vi "Write txt.vi"(8 "error in":errorcluster, 11 "IN String":string) -> (0 "error out":errorcluster, 3 "out":string)   [LabVIEW 2009]
uses:
  Global/Global 1.vi
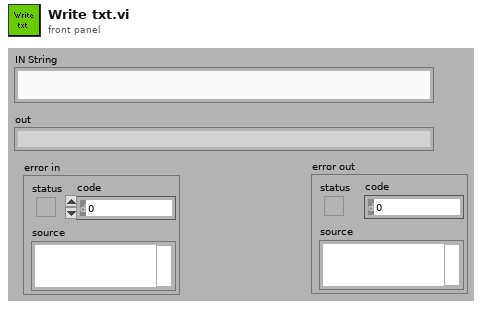
[diagram p1: front panel]
types:
  T1 = enum16{"open", "replace", "create", "open or create", "replace or create", "replace or create with confirmation"}
  T2 = cluster{"serial number":string, "Part number":string, "Revision letter ":string, "Revision counter":string, "Manufature":string, "Year Week":string}
  T3 = cluster{".128 file":path, "Appliction firmware file":path, "Data file":path, "Txt path":path, "EXCEL path":path}
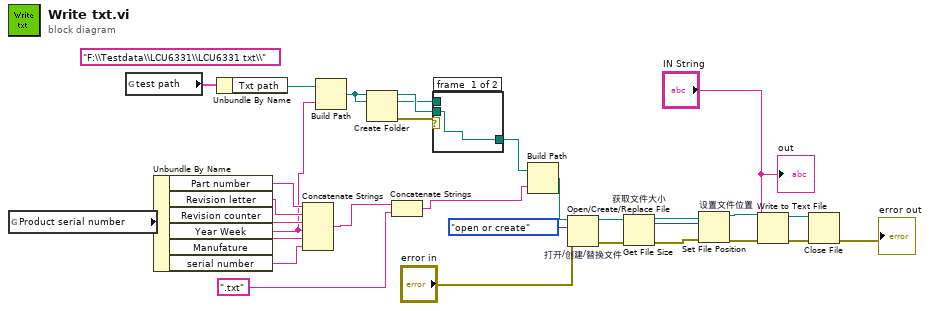
[diagram p0: block diagram]
diagram:
  (unwired) "F:\\Testdata\\LCU6331\\LCU6331 txt\\" ("string")
  n1 = global read "Global 1.vi" "Product serial number"() -> (w16:T2)
  n2 = global read "Global 1.vi" "test path"() -> (w2:T3)
  n3 = Unbundle By Name(w16) -> ("Part number"=w15:string, "Revision letter"=w14:string, "Revision counter"=w13:string, "Year Week"=w9:string, "Manufature"=w12:string, "serial number"=w11:string)
  n4 = Unbundle By Name(w2) -> ("Txt path"=w1:path)
  n5 = Concatenate Strings(w15, w14, w13, w9, w12, w11) -> (w10:string)
  n6 = Build Path(base path=w1, name or relative path=w9) -> (appended path=w6:path)
  n7 = Create Folder(path (use dialog)=w6) -> (created path=w8:path, error out=w7:errorcluster)  [unwired: 1 in, 2 out]
  n8 = Concatenate Strings(w10, ".txt") -> (w4:string)
  n9 = case shown="Error" w7 {
    tunnel: w8 -> [w31 _]
    tunnel: [w31 w32] -> w5
    tunnel: w6 -> [_ w32]
    frame #0 {
    }
    frame #1 {
    }
  }
  n10 = Build Path(base path=w5, name or relative path=w4) -> (appended path=w3:path)
  n11 = Open/Create/Replace File "打开/创建/替换文件"(file path (use dialog)=w3, error in="error in", operation (0:open)=T1."open or create" ("操作(0:open)")) -> (refnum out=w27:refnum<file>, error out=w25:errorcluster)  [unwired: 4 out]
  n12 = Get File Size "获取文件大小"(file=w27, error in=w25) -> (refnum out=w28:refnum<file>, size (in bytes)=w22:i64, 0:w29:errorcluster)
  n13 = Set File Position "设置文件位置"(offset (in bytes) (0)=w22, refnum=w28, error in=w29) -> (refnum out=w26:refnum<file>, error out=w24:errorcluster)  [unwired: 1 in]
  n14 = Write to Text File(file (use dialog)=w26, text="IN String", error in=w24) -> (refnum out=w18:refnum<file>, error out=w19:errorcluster)  [unwired: 2 out]
  n15 = Close File(refnum=w18, error in=w19) -> (error out=→"error out":errorcluster)  [unwired: 1 out]
  "out" <- "IN String"
